vi "Cursor Set.vi"(8 "error in (no error)":errorcluster caption="错误输入（无错误）", 10 "Cursor":enum16{"Idle", "Busy"}(ring), 11 "Nested in":refnum<class "RefNums and UICtrl.lvclass">) -> (0 "error out":errorcluster caption="错误输出", 3 "Nested out":refnum<class "RefNums and UICtrl.lvclass">)   [LabVIEW 2020, in "RefNums and UICtrl.lvclass"]
uses:
  RefNums and UICtrl.lvclass
  RefNums and UICtrl.lvclass/RefNums and UICtrl.ctl
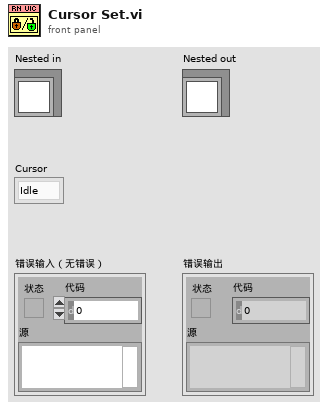
[diagram p1: front panel]
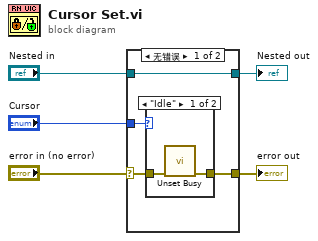
[diagram p0: block diagram]
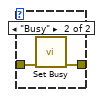
[diagram p2: hidden frame]
diagram:
  n1 = case shown="无错误" "error in (no error)" {
    selector: "error in (no error)" -> [w8 w15]
    tunnel: [w6 w15] -> w4
    tunnel: [w9 w14] -> w2
    tunnel: "Nested in" -> [w9 w14]
    tunnel: "Cursor" -> [w7 _]
    frame No Error {
      n2 = case shown="\"Idle\"" w7 {
        tunnel: w8 -> [w11 w13]
        tunnel: [w10 w12] -> w6
        frame "Idle" {
          n3 = call <vilib>:"Unset Busy.vi"("error in (no error)"=w11) -> ("error out"=w10:errorcluster)  [unwired: 10 in]
        }
        frame "Busy" {
          n4 = call <vilib>:"Set Busy.vi"("error in (no error)"=w13) -> ("error out"=w12:errorcluster)  [unwired: 9 in, 1 out]
        }
      }
    }
    frame Error {
    }
  }
  "error out" <- w4
  "Nested out" <- w2
